vi "Remove Nested Model.vi"(10 "Nested Model Enqueuer":refnum<class "Message Enqueuer.lvclass">, 11 "IModel in":refnum<class "IModel.lvclass">) -> (2 "None Remaining?":bool, 3 "IModel out":refnum<class "IModel.lvclass">)   [LabVIEW 2019, in "IModel.lvlib" / "IModel.lvclass"]
uses:
  <vilib>/gpm_packages/@cs/mva-core/Source/IModel/IModel/IModel.lvclass
  <vilib>/ActorFramework/Message Enqueuer/Message Enqueuer.lvclass
  <vilib>/gpm_packages/@cs/mva-core/Source/IModel/IModel/IModel.lvclass/IModel.ctl
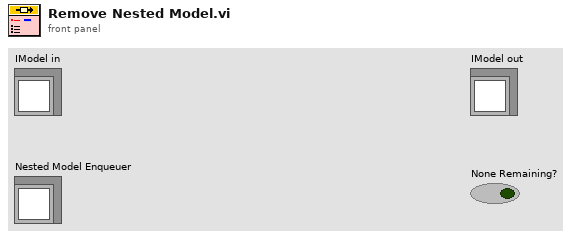
[diagram p1: front panel]
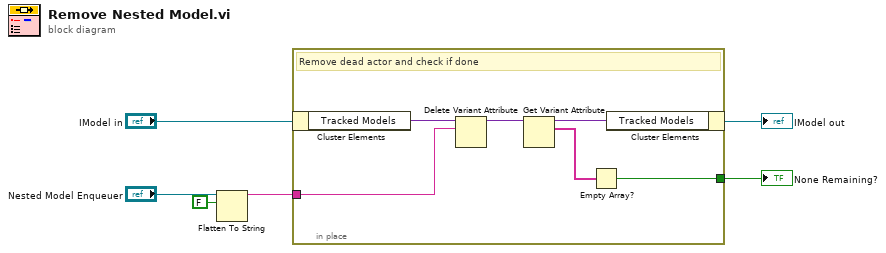
[diagram p0: block diagram]
diagram:
  n1 = Flatten To String(anything="Nested Model Enqueuer", prepend array or string size? (T)=FALSE) -> (data string=w4:string)  [unwired: 2 in, 2 out]
  n2 = in-place {
    in-place-border: w4 -> [w11]
    in-place-border: [w7] -> w5
    # "Remove dead actor and check if done"
    n3 = in-place-cluster #1("IModel in") -> ("Tracked Models"=w12:variant)
    n4 = Delete Variant Attribute(6:w11, 7:w12) -> (3:w10:variant)  [unwired: 1 in, 2 out]
    n5 = Get Variant Attribute(Variant=w10) -> (duplicate Variant=w9:variant, names=w8:string[])  [unwired: 3 in, 2 out]
    n6 = Empty Array?(array=w8) -> (empty?=w7:bool)
    n7 = in-place-cluster #1("Tracked Models"=w9) -> (→"IModel out":refnum<class "IModel.lvclass">)
  }
  "None Remaining?" <- w5
